vi "selfConfigRead.vi"(8 "error in":errorcluster) -> (0 "error out":errorcluster, 2 "configPath":path, 3 "refDes":string)   [LabVIEW 2024]
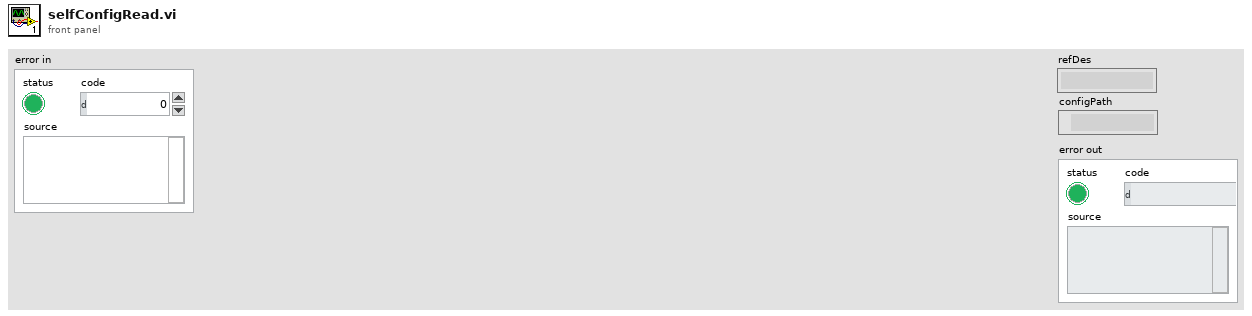
[diagram p1: front panel]
types:
  T1 = cluster{"Sheet Data[0]":cluster{"Array":string[][]}}
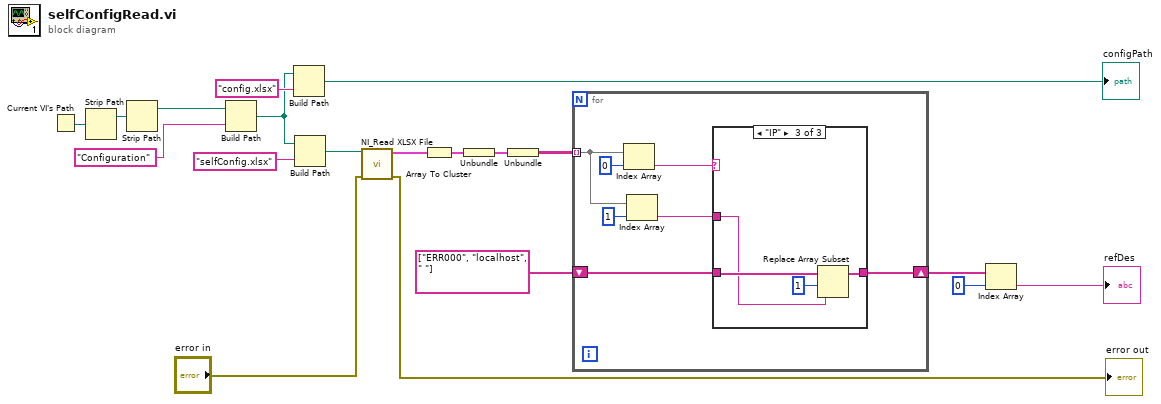
[diagram p0: block diagram]
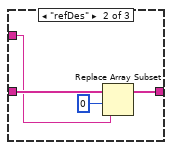
[diagram p3: hidden frame]
diagram:
  n1 = Current VI's Path() -> (path=w12:path)
  n2 = Strip Path(path=w12) -> (stripped path=w13:path)  [unwired: 1 out]
  n3 = Strip Path(path=w13) -> (stripped path=w3:path)  [unwired: 1 out]
  n4 = Build Path(base path=w3, name or relative path="Configuration") -> (appended path=w1:path)
  n5 = Build Path(base path=w1, name or relative path="config.xlsx") -> (appended path=→"configPath":path)
  n6 = Build Path(base path=w1, name or relative path="selfConfig.xlsx") -> (appended path=w18:path)
  n7 = call "NI_Read XLSX File.vi"("error in"="error in", "XLSX File"=w18) -> ("error out"=→"error out":errorcluster, "Sheet Data"=w17:cluster{"Array":string[][]}[])  [unwired: 7 in, 1 out]
  n8 = Array To Cluster(array=w17) -> (cluster=w16:T1)
  n9 = Unbundle(w16) -> ("Sheet Data[0]"=w15:cluster{"Array":string[][]})
  n10 = Unbundle(w15) -> ("Array"=w14:string[][])
  n11 = for {
    tunnel: w14 -> [w24] mode=indexing
    shift-right: [w21] -> w10
    shift-left: string[] ["ERR000", "localhost", " "] -> [w22]
    n12 = Index Array(array=w24, index=0) -> (element=w23:string)
    n13 = Index Array(array=w24, index=1) -> (element=w20:string)
    n14 = case shown="\"IP\"" w23 {
      tunnel: w22 -> [w27 w31 w34]
      tunnel: [w27 w30 w32] -> w21
      tunnel: w20 -> [_ w28 w33]
      frame Default {
      }
      frame "refDes" {
        n15 = Replace Array Subset(array=w31, new element=w28, index=0) -> (w30:string[])
      }
      frame "IP" {
        n16 = Replace Array Subset(array=w34, new element=w33, index=1) -> (w32:string[])
      }
    }
  }
  n17 = Index Array(array=w10, index=0) -> (element=→"refDes":string)
